vi "Set ROI(SubVI).vi"(10 "Nr of objects":dbl, 11 "Numeric":dbl) -> (3 "Cluster":cluster{dbl, dbl, dbl, dbl, dbl})   [LabVIEW 2014]
uses:
  Global.vi
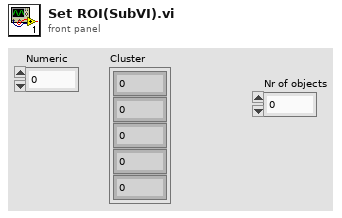
[diagram p1: front panel]
types:
  T1 = cluster{"Numeric":dbl, "Numeric":dbl, "Numeric":dbl, "Numeric":dbl}
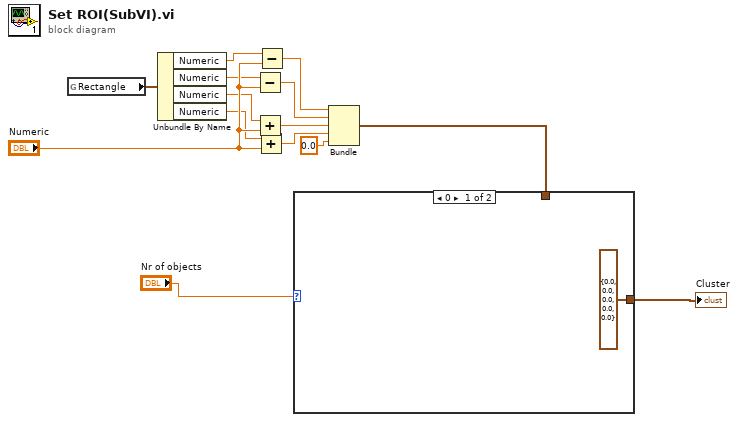
[diagram p0: block diagram]
diagram:
  n1 = global read "Global.vi" "Rectangle"() -> (w4:T1)
  n2 = Unbundle By Name(w4) -> ("Numeric"=w6:dbl, "Numeric"=w8:dbl, "Numeric"=w10:dbl, "Numeric"=w12:dbl)
  n3 = Subtract(x=w8, y="Numeric") -> (x-y=w9:dbl)
  n4 = Add(x=w10, y="Numeric") -> (x+y=w11:dbl)
  n5 = Add(x=w12, y="Numeric") -> (x+y=w13:dbl)
  n6 = Subtract(x=w6, y="Numeric") -> (x-y=w7:dbl)
  n7 = Bundle(w7, w9, w11, w13, 0.0) -> (w3:cluster{dbl, dbl, dbl, dbl, dbl})  [unwired: 1 in]
  n8 = case shown="0" "Nr of objects" {
    tunnel: w3 -> [_ w16]
    tunnel: [cluster{dbl, dbl, dbl, dbl, dbl} {0.0, 0.0, 0.0, 0.0, 0.0} w16] -> w1
    frame 0 {
    }
    frame 1, Default {
    }
  }
  "Cluster" <- w1
